vi "TEMPLATE_Constructor.vi"(8 "Error In":errorcluster, 11 "Post-Bundled Subclass":refnum<class "LQObject.lvclass">) -> (0 "Error Out":errorcluster, 3 "%TYPE% Out":refnum<class "LQObject.lvclass">)   [LabVIEW 2013, in "Template.lvlib" / "LQObject.lvclass"]
uses:
  LQObject.lvclass
  LQIdentity/LQIdentity.lvclass
  LQWidgetEngine/LQWidgetEngine.lvclass
  LQWidgetEngine/Internal/LQIdentity Registry Action.ctl
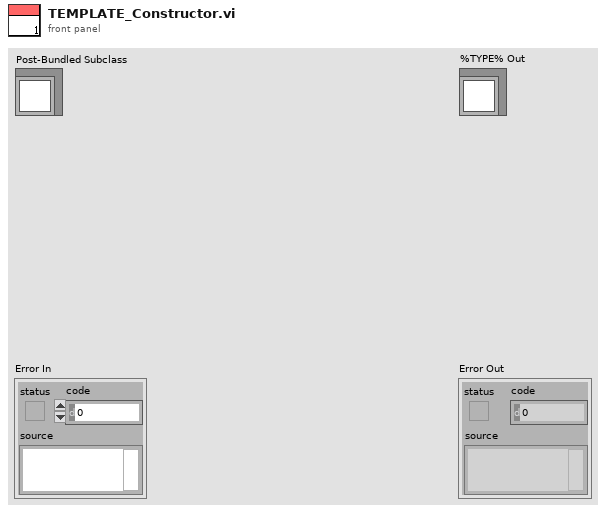
[diagram p1: front panel]
types:
  T1 = typedef "Template.lvlib/LQWidgetEngine.lvclass/LQIdentity Registry Action.ctl" = enum16{"Init", "Register LQIdentity", "Get LQIdentity Info", "Deregister LQIdentity"}
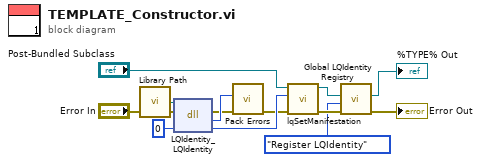
[diagram p0: block diagram]
diagram:
  n1 = call "Library Path.vi"() -> ("Library Path"=w10:path)
  n2 = dll-call lib="?" fn="LQIdentity_LQIdentity"(path in=w10, error in="Error In", "_instance"=u64 0) -> (error out=w8:errorcluster, "errorCode"=w9:i32, "_instance"=w11:u64)  [unwired: 1 in, 1 out]
  n3 = call "Pack Errors.vi"("Error In"=w8, "Error Code"=w9) -> ("Error Out"=w7:errorcluster)  [unwired: 9 in]
  n4 = call "lqSetManifestation.vi"("Error In"=w7, "Manifestation"=w11, "LQIdentity in"="Post-Bundled Subclass") -> ("Error Out"=w5:errorcluster, "LQIdentity out"=w6:refnum<class "LQObject.lvclass">)  [unwired: 7 in]
  n5 = call "Global LQIdentity Registry.vi"("Error In"=w5, "Registry Action"=LQIdentity_Registry_Action."Register LQIdentity", "LQIdentity Info In"=w6) -> ("Error Out"=→"Error Out":errorcluster, "LQIdentity Info Out"=→"%TYPE% Out":refnum<class "LQObject.lvclass">)  [unwired: 7 in]
